vi "Init_Sim.vi"(10 "SimAlg.lvclass":refnum<class "PrllPerElmnt.lvclass">, 11 "QuSim in":refnum<class "QuSim.lvclass">) -> (3 "QuSim out":refnum<class "QuSim.lvclass">)   [LabVIEW 2020, in "QuSim.lvclass"]
uses:
  QuSim.lvclass
  SimAlg/PrllPerElement/PrllPerElmnt.lvclass
  QuWire/QuWire.lvclass
  C:/Users/morte/OneDrive/LabVIEW/Quantum Circuit Simulator/VIPM/QuVI 2020/QuSim/QuSim.lvclass
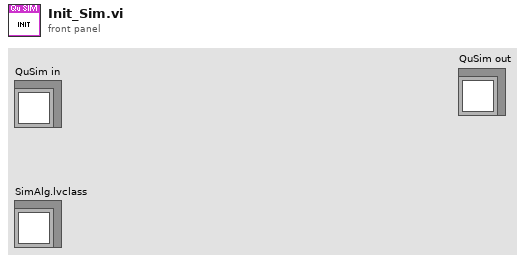
[diagram p1: front panel]
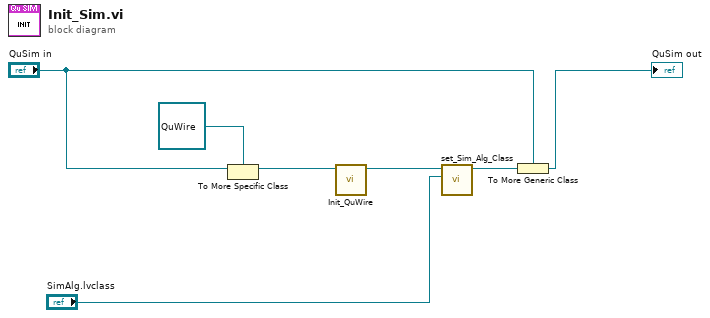
[diagram p0: block diagram]
diagram:
  n1 = To More Specific Class(target class=refnum<class "QuWire.lvclass"> refnum ("Wire.lvclass"), reference="QuSim in") -> (specific class reference=w4:refnum<class "QuWire.lvclass">)  [unwired: 1 in, 1 out]
  n2 = call "Init_QuWire.vi"("QuWire in"=w4) -> ("QuWire out"=w3:refnum<class "QuWire.lvclass">)  [unwired: 9 in, 1 out]
  n3 = call "set_Sim_Alg_Class.vi"("SimAlg.lvclass"="SimAlg.lvclass", "QuWire in"=w3) -> ("QuWire out"=w2:refnum<class "QuWire.lvclass">)  [unwired: 8 in, 1 out]
  n4 = To More Generic Class(target class="QuSim in", reference=w2) -> (generic class reference=→"QuSim out":refnum<class "QuSim.lvclass">)
